vi "Frame.CheckErrors.vi"(7 "Existing PIDs":string[](array[string]), 8 "error in (no error)":errorcluster, 9 "ID":refnum<vi>, 10 "Name":refnum<vi>, 11 "Listbox":refnum<vi>) -> (0 "error out":errorcluster, 2 "Error Type":string, 3 "Error?":bool)   [LabVIEW 2015, in "Diagnostics Addon System Explorer.lvlib"]
uses:
  Diagnostics Addon System Explorer.lvlib
  Shared/Types/XNET.Frame.ctl
  Shared/SubVIs/GUID Lookup.vi
  <vilib>/xnet/xnet.llb/XNET Database Create (Cluster).vi
  <vilib>/xnet/xnet.llb/XNET Database Delete (Cluster).vi
  <vilib>/xnet/xnet.llb/XNET Database Close (Database).vi
  Shared/Diagnostics Addon Shared.lvlib
  <resource>/objmgr/xnet.rc
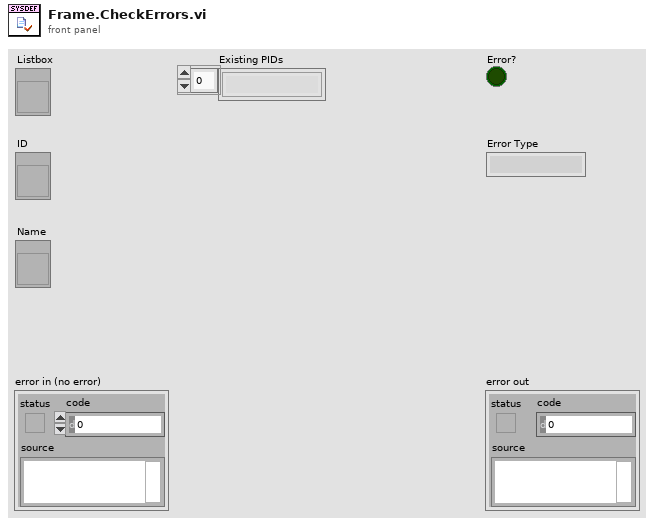
[diagram p1: front panel]
types:
  T1 = enum16{"CheckSignalNames", "CheckBits", "CheckName"}[]
  T2 = typedef "Diagnostics Addon Shared.lvlib/Signal.ctl" = cluster{"Start Bit":u8, "Length":u8, "Scaling Factor":dbl, "Scaling Offset":dbl, "Minimum":dbl, "Maximum":dbl, "Data Type":u32, "Byte Order":u32, "Default Value":dbl, "Name":string, "Units":string, "Description":string}
  T3 = typedef "Diagnostics Addon Shared.lvlib/XNET.Frame.ctl" = cluster{"Frame name":string, "Identifier":u32, "Payload Length":u32, "Timing Type":u32, "Transmit Time":dbl, "Extended Identifier?":bool, "Comment":string}
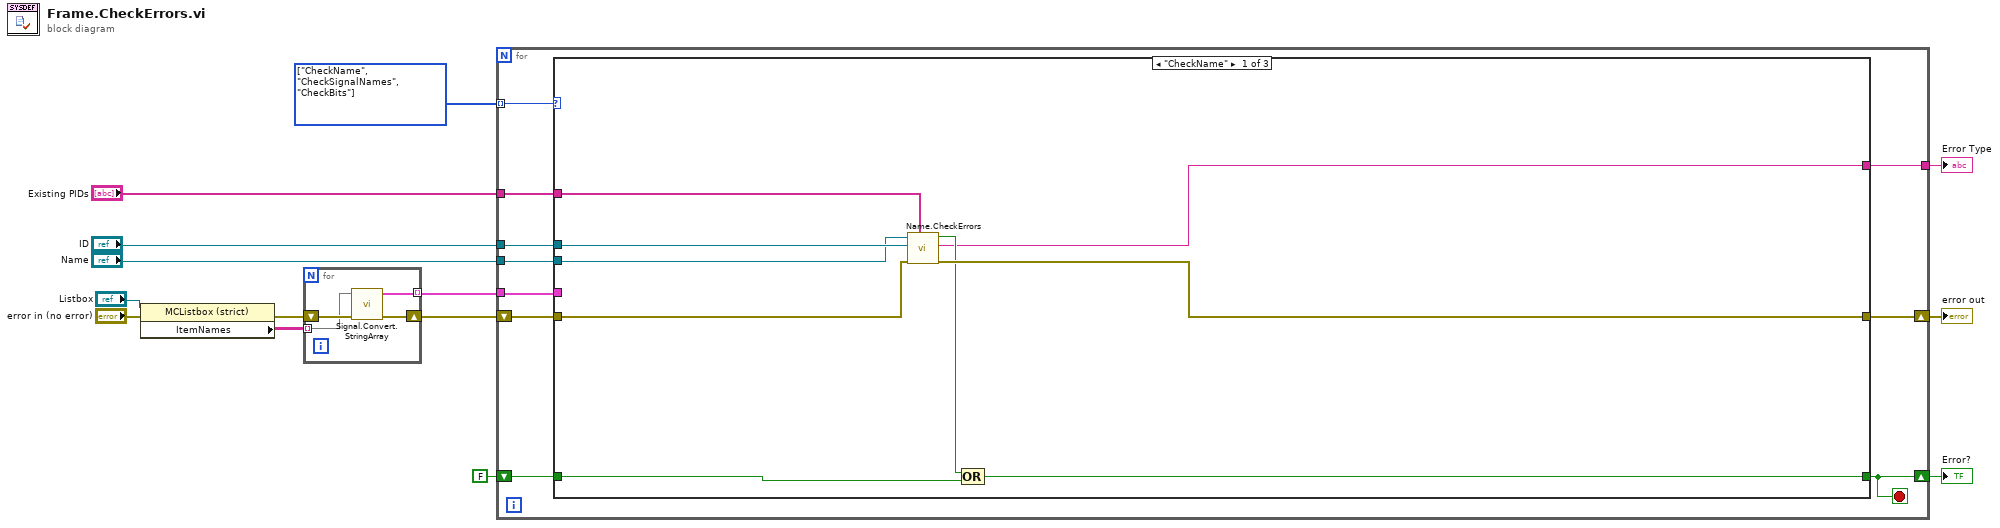
[diagram p0: block diagram]
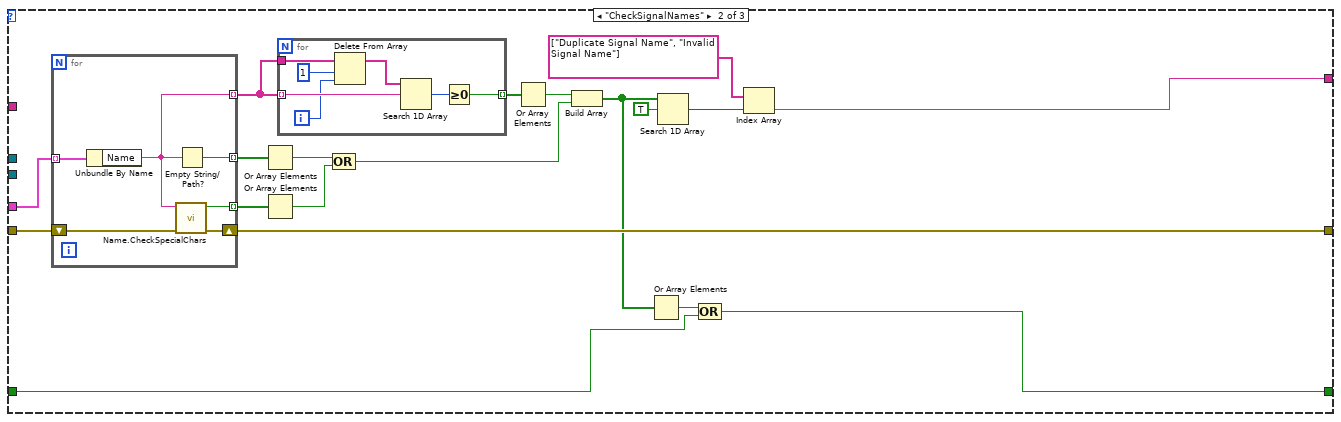
[diagram p2: hidden frame]
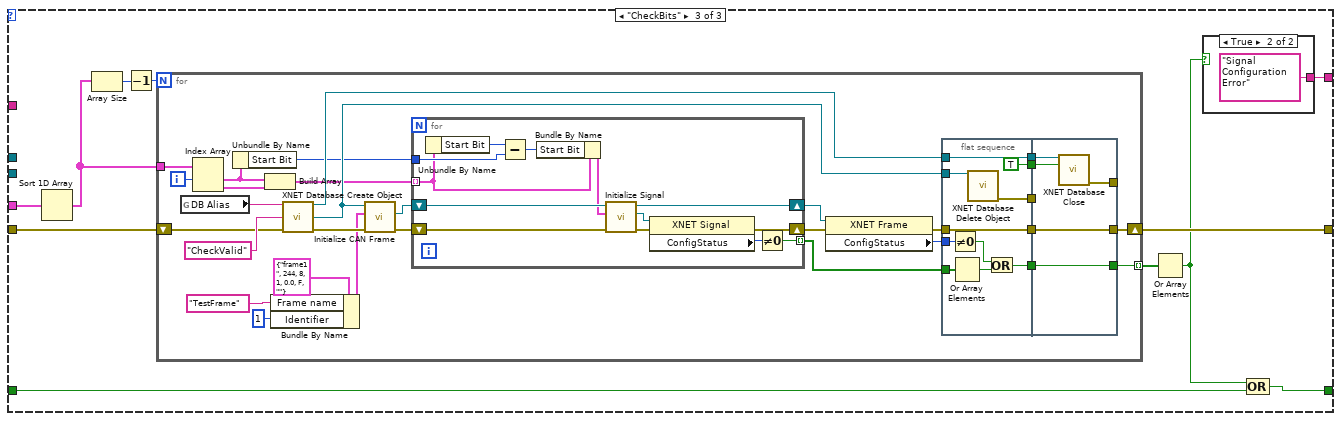
[diagram p3: hidden frame]
diagram:
  w10 = T1 [enum."CheckName", enum."CheckSignalNames", enum."CheckBits"] items=["CheckSignalNames", "CheckBits", "CheckName"]
  n1 = property class="MCListbox (strict)"(reference="Listbox", error in="error in (no error)") -> (error out=w13:errorcluster, "ItemNames"=w14:string[][])  [unwired: 1 out]
  n2 = for {
    shift-right: [w17] -> w9
    shift-left: w13 -> [w18]
    tunnel: w14 -> [w16] mode=indexing
    tunnel: [w15] -> w8 mode=indexing
    n3 = call "Signal.Convert.StringArray.vi"("error in (no error)"=w18, "Signal Parameters"=w16) -> ("error out"=w17:errorcluster, "Signal Parameters"=w15:T2)  [unwired: 8 in]
  }
  n4 = for {
    tunnel: w10 -> [w28] mode=indexing
    shift-right: [w25] -> w5
    shift-left: w9 -> [w24]
    tunnel: w8 -> [w27]
    shift-right: [w19] -> w6
    shift-left: FALSE -> [w26]
    tunnel: "Existing PIDs" -> [w23]
    tunnel: "Name" -> [w22]
    tunnel: "ID" -> [w21]
    tunnel: [w20] -> w1
    stop <- w19 stop-if-true
    n5 = case shown="\"CheckName\"" w28 {
      tunnel: w27 -> [_ w56 w74]
      tunnel: [w34 w45 w79] -> w19
      tunnel: w26 -> [w35 w44 w80]
      tunnel: [w36 w49 w73] -> w25
      tunnel: w24 -> [w37 w50 w70]
      tunnel: w23 -> [w31 _ _]
      tunnel: w22 -> [w29 _ _]
      tunnel: w21 -> [w30 _ _]
      tunnel: [w32 w38 w72] -> w20
      frame "CheckName" {
        n6 = call "Name.CheckErrors.vi"("Existing Frames"=w31, "error in (no error)"=w37, "ID"=w30, "Name"=w29) -> ("error out"=w36:errorcluster, "Error"=w32:string, "Error?"=w33:bool)  [unwired: 5 in]
        n7 = Compound Arithmetic op=OR(w33, w35) -> (w34:bool)
      }
      frame "CheckSignalNames" {
        n8 = for {
          tunnel: w56 -> [w69] mode=indexing
          tunnel: [w66] -> w55 mode=indexing
          tunnel: [w68] -> w54 mode=indexing
          tunnel: [w67] -> w51 mode=indexing
          shift-right: [w64] -> w49
          shift-left: w50 -> [w65]
          n9 = Unbundle By Name(w69) -> ("Name"=w68:string)
          n10 = call "Name.CheckSpecialChars.vi"("error in"=w65, "Signal Name"=w68) -> ("error out"=w64:errorcluster, "Special Character?"=w67:bool)  [unwired: 8 in]
          n11 = Empty String/Path?(string/path=w68) -> (empty?=w66:bool)
        }
        n12 = Or Array Elements(Boolean array=w55) -> (logical OR=w42:bool)
        n13 = Or Array Elements(Boolean array=w51) -> (logical OR=w43:bool)
        n14 = for {
          tunnel: w54 -> [w58]
          tunnel: w54 -> [w63] mode=indexing
          tunnel: [w61] -> w53 mode=indexing
          i -> [w59]
          n15 = Delete From Array(array=w58, length=1, index=w59) -> (array with subset deleted=w57:string[])  [unwired: 1 out]
          n16 = Search 1D Array(1D array=w57, element=w63) -> (index of element=w62:i32)  [unwired: 1 in]
          n17 = Greater Or Equal To 0?(x=w62) -> (x >= 0?=w61:bool)
        }
        n18 = Compound Arithmetic op=OR(w42, w43) -> (w41:bool)
        n19 = Or Array Elements(Boolean array=w53) -> (logical OR=w52:bool)
        n20 = Build Array(w52, w41) -> (w47:bool[])
        n21 = Or Array Elements(Boolean array=w47) -> (logical OR=w46:bool)
        n22 = Search 1D Array(1D array=w47, element=TRUE) -> (index of element=w40:i32)  [unwired: 1 in]
        n23 = Compound Arithmetic op=OR(w46, w44) -> (w45:bool)
        n24 = Index Array(array=string[] ["Duplicate Signal Name", "Invalid Signal Name"], index=w40) -> (element=w38:string)
      }
      frame "CheckBits" {
        n25 = Sort 1D Array(array=w74) -> (sorted array=w78:T2[])
        n26 = Array Size(array=w78) -> (size(s)=w75:i32)
        n27 = Decrement(x=w75) -> (x-1=w76:i32)
        n28 = for {
          N: w76 -> [_]
          tunnel: [w82] -> w77 mode=indexing
          tunnel: w78 -> [w94]
          shift-right: [w93] -> w73
          shift-left: w70 -> [w92]
          i -> [w91]
          n29 = global read "GUID Lookup.vi" "DB Alias"() -> (w98:string)
          n30 = Index Array(array=w94, index #1=w91) -> (element #1=w88:T2, element #2=w90:T2)  [unwired: 1 in]
          n31 = Unbundle By Name(w88) -> ("Start Bit"=w87:u8)
          n32 = Build Array(w88, w90) -> (w89:T2[])
          n33 = Bundle By Name(cluster=T3 {"Frame name"="frame1", "Identifier"=244, "Payload Length"=8, "Timing Type"=1, "Transmit Time"=0.0, "Extended Identifier?"=FALSE, "Comment"=""} ("CAN Frame"), "Frame name"="TestFrame" ("cluster name"), "Identifier"=u32 1) -> (w101:T3)
          n34 = call-poly <vilib>:"XNET Database Create Object.vi"("database in"=w98, "cluster name"="CheckValid", "error in (no error)"=w92) -> ("database out"=w95:refnum<k21>, "cluster out"=w96:refnum<k21>, "error out"=w102:errorcluster)  [unwired: 10 in]
          n35 = call "Initialize CAN Frame.vi"("error in"=w102, "CAN Frame"=w101, "cluster in"=w96) -> ("error out"=w105:errorcluster, "frame out"=w106:refnum<k21>)  [unwired: 6 in, 1 out]
          n36 = for {
            shift-right: [w132] -> w107
            shift-left: w105 -> [w138]
            tunnel: w89 -> [w127] mode=indexing
            tunnel: [w133] -> w85 mode=indexing
            shift-right: [w131] -> w99
            shift-left: w106 -> [w137]
            tunnel: w87 -> [w129]
            n37 = Unbundle By Name(w127) -> ("Start Bit"=w130:u8)
            n38 = Subtract(x=w130, y=w129) -> (x-y=w128:u8)
            n39 = Bundle By Name(cluster=w127, "Start Bit"=w128) -> (w126:T2)
            n40 = call "Initialize Signal.vi"("error in"=w138, "Signal"=w126, "frame in"=w137) -> ("error out"=w135:errorcluster, "signal out"=w136:refnum<k21>, "frame out"=w131:refnum<k21>)  [unwired: 6 in]
            n41 = property class="XNET Signal"(reference=w136, error in=w135) -> (error out=w132:errorcluster, "ConfigStatus"=w134:i32)  [unwired: 1 out]
            n42 = Not Equal To 0?(x=w134) -> (x != 0?=w133:bool)
          }
          n43 = property class="XNET Frame"(reference=w99, error in=w107) -> (error out=w84:errorcluster, "ConfigStatus"=w86:i32)  [unwired: 1 out]
          n44 = flat-sequence {
            tunnel: w84 -> [w119]
            tunnel: w96 -> [w120]
            tunnel: w95 -> [w118]
            tunnel: [w119] -> w110
            tunnel: [w118] -> w109
            tunnel: [w117] -> w108
            tunnel: w86 -> [w114]
            tunnel: w85 -> [w113]
            tunnel: [w112] -> w83
            tunnel: [TRUE ("close all? (true)")] -> w81
            tunnel: w110 -> [w125]
            tunnel: w109 -> [w124]
            tunnel: w108 -> [_]
            tunnel: w83 -> [w123]
            tunnel: [w125] -> w93
            tunnel: [w123] -> w82
            tunnel: [w122] -> _
            tunnel: w81 -> [w121]
            frame #0 {
              n45 = Not Equal To 0?(x=w114) -> (x != 0?=w116:bool)
              n46 = Or Array Elements(Boolean array=w113) -> (logical OR=w115:bool)
              n47 = call-poly <vilib>:"XNET Database Delete Object.vi"("cluster in"=w120) -> ("error out"=w117:errorcluster)  [unwired: 14 in]
              n48 = Or(x=w116, y=w115) -> (x .or. y?=w112:bool)
            }
            frame #1 {
              n49 = call-poly <vilib>:"XNET Database Close.vi"("database in"=w124, "close all? (true)"=w121) -> ("error out"=w122:errorcluster)  [unwired: 13 in]
            }
          }
        }
        n50 = Or Array Elements(Boolean array=w77) -> (logical OR=w71:bool)
        n51 = case shown="True" w71 {
          tunnel: [_ "Signal Configuration Error"] -> w72
          frame False {
          }
          frame True {
          }
        }
        n52 = Compound Arithmetic op=OR(w71, w80) -> (w79:bool)
      }
    }
  }
  "Error?" <- w6
  "error out" <- w5
  "Error Type" <- w1
